vi "CreatePrivateEvents.vi"(8 "error in (no error)":errorcluster, 11 "CircularBuffer":refnum<class "CircularBuffer.lvclass">) -> (0 "error out":errorcluster, 3 "CircularBuffer out":refnum<class "CircularBuffer.lvclass">)   [LabVIEW 2015, in "CircularBuffer.lvclass"]
doc: "JKI State Machine Objects (SMO) 1.0.2.13\nJKI - JKI\nCopyright (c) 2016, JKI"
uses:
  CircularBuffer.lvclass
  CircularBuffer.lvclass/CircularBuffer.ctl
  Typedefs/NewBufferSize--Cluster.ctl
  Typedefs/BufferSize.ctl
  Typedefs/PrivateEvents--CircularBuffer.GetElement.ctl
  <vilib>/JKI/JKI SMO/SMO/SMO.lvclass
panel:
  # "For instructions on how to use the JKI State Machine Objects, examples and video tutorials, visit:\nhttp://jki.net/state-machine-objects/\n\nJKI State Machine Objects™\nhttp://jki.net/state-machine-objects/\nCopyright (C) 2005-2015, JKI <info@jki.net>\nALL RIGHTS RESERVED"
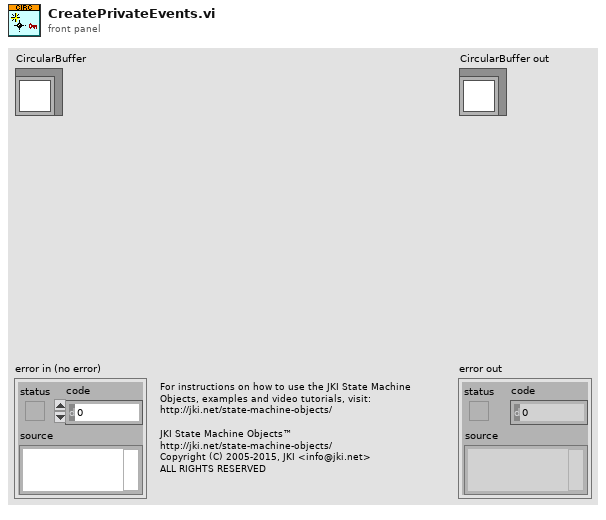
[diagram p1: front panel]
types:
  T1 = typedef "CircularBuffer.lvclass/PrivateData--Ref.ctl" = refnum<data-value>
  T2 = typedef "CircularBuffer.lvclass/PrivateEvents--CircularBuffer.GetElement.ctl" = u32
  T3 = typedef "CircularBuffer.lvclass/NewBufferSize--Cluster.ctl" = cluster{"BufferSize":T4}
  T4 = typedef "CircularBuffer.lvclass/BufferSize.ctl" = u32
  T5 = typedef "CircularBuffer.lvclass/PrivateData--Cluster.ctl" = cluster{"Public Events":T6, "Protected Events":T7, "Private Events":T8, "BufferSize":T4, "CurrentElement":u32}
  T6 = typedef "CircularBuffer.lvclass/PublicEvents--Cluster.ctl" = cluster{"Buffer Resize Event":refnum<user-event>}
  T7 = typedef "CircularBuffer.lvclass/ProtectedEvents--Cluster.ctl" = cluster{"placeholder":refnum<user-event>}
  T8 = typedef "CircularBuffer.lvclass/PrivateEvents--Cluster.ctl" = cluster{"New Value":refnum<user-event>, "GetElement":refnum<user-event>}
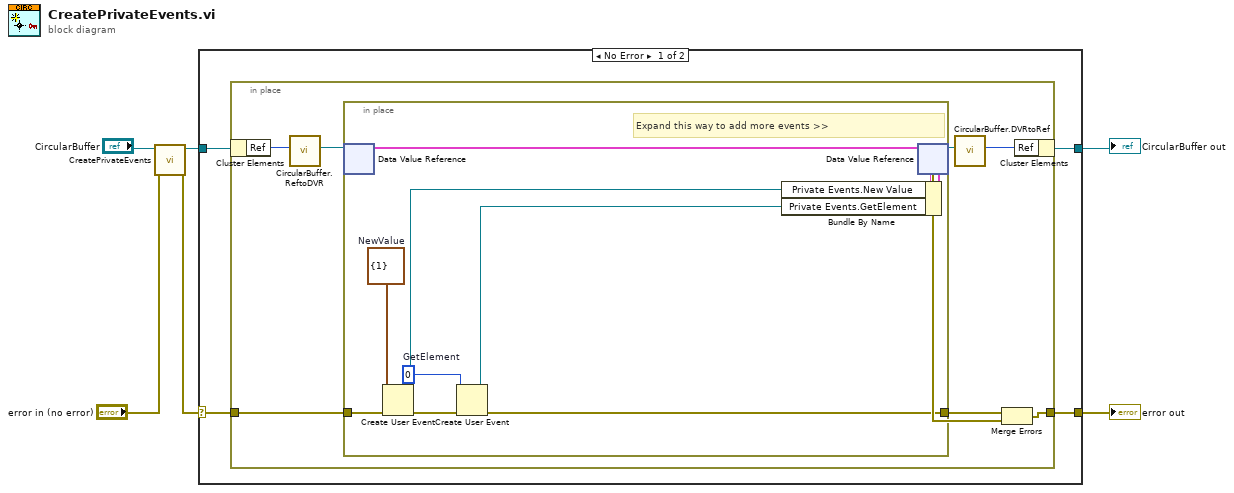
[diagram p0: block diagram]
diagram:
  n1 = call-parent "CreatePrivateEvents.vi"("error in (no error)"="error in (no error)", "SMO"="CircularBuffer") -> ("error out"=w5:errorcluster, "SMO out"=w6:refnum<class "CircularBuffer.lvclass">)  [unwired: 8 in]
  n2 = case shown="No Error" w5 {
    selector: w5 -> [w8 w29]
    tunnel: [w7 w29] -> w1
    tunnel: [w9 w28] -> w3
    tunnel: w6 -> [w10 w28]
    frame No Error {
      n3 = in-place {
        in-place-border: w8 -> [w18]
        in-place-border: [w15] -> w7
        n4 = in-place-cluster #1(w10) -> ("Ref"=w14:u32)
        n5 = call "CircularBuffer.ReftoDVR.vi"("Ref"=w14) -> ("Ref"=w13:T1)  [unwired: 10 in]
        n6 = in-place {
          in-place-border: w18 -> [w25]
          in-place-border: [w21] -> w17
          w20 = T2 0  # GetElement
          w22 = T3 {"BufferSize"=1}  # NewValue
          # "Expand this way to add more events >>"
          n7 = in-place-dvr #2(w13) -> (w24:T5)  [unwired: 1 out]
          n8 = Create User Event(user event datatype=w22, error in=w25) -> (user event=w23:refnum<user-event>, error out=w26:errorcluster)
          n9 = Create User Event(user event datatype=w20, error in=w26) -> (user event=w19:refnum<user-event>, error out=w21:errorcluster)
          n10 = Bundle By Name(cluster=w24, "Private Events.New Value"=w23, "Private Events.GetElement"=w19) -> (w27:T5)
          n11 = in-place-dvr #2(w27) -> (w12:T1, w16:errorcluster)
        }
        n12 = call "CircularBuffer.DVRtoRef.vi"("Ref"=w12) -> ("Ref"=w11:u32)  [unwired: 10 in]
        n13 = Merge Errors(w17, w16) -> (w15:errorcluster)
        n14 = in-place-cluster #1("Ref"=w11) -> (w9:refnum<class "CircularBuffer.lvclass">)
      }
    }
    frame Error {
    }
  }
  "error out" <- w1
  "CircularBuffer out" <- w3
